vi "Init.vi"(8 "error in":errorcluster, 11 "XML Editor GUI in":refnum<class "XML Editor GUI.lvclass">) -> (0 "error out":errorcluster, 3 "XML Editor GUI out":refnum<class "XML Editor GUI.lvclass">)   [LabVIEW 2014, in "XML Editor GUI.lvclass"]
uses:
  XML Editor GUI.lvclass
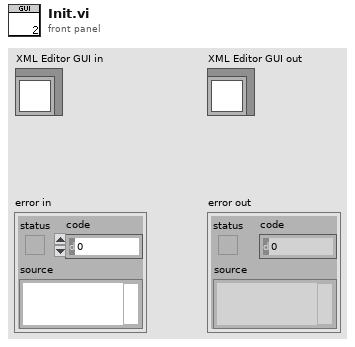
[diagram p1: front panel]
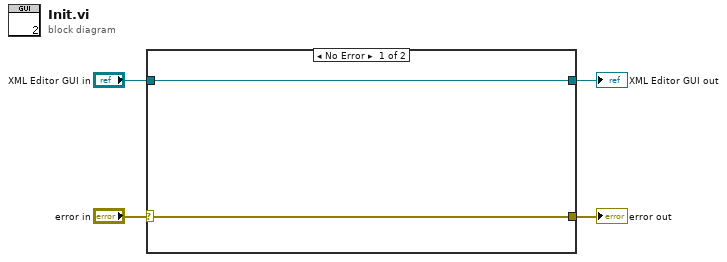
[diagram p0: block diagram]
diagram:
  n1 = case shown="No Error" "error in" {
    selector: "error in" -> [w5 w8]
    tunnel: [w5 w8] -> w3
    tunnel: [w6 w7] -> w1
    tunnel: "XML Editor GUI in" -> [w6 w7]
    frame No Error {
    }
    frame Error {
    }
  }
  "error out" <- w3
  "XML Editor GUI out" <- w1
